vi "Set Geometry.vi"(0 "reference in":refnum<class "Manipulator.lvclass">, 5 "Lengths.a":dbl, 7 "Lengths.b":dbl, 9 "Lengths.c":dbl, 11 "error in (no error)":errorcluster) -> (4 "reference out":refnum<class "Manipulator.lvclass">, 15 "error out":errorcluster)   [LabVIEW 2014, in "Manipulator.lvclass"]
uses:
  Manipulator.lvclass
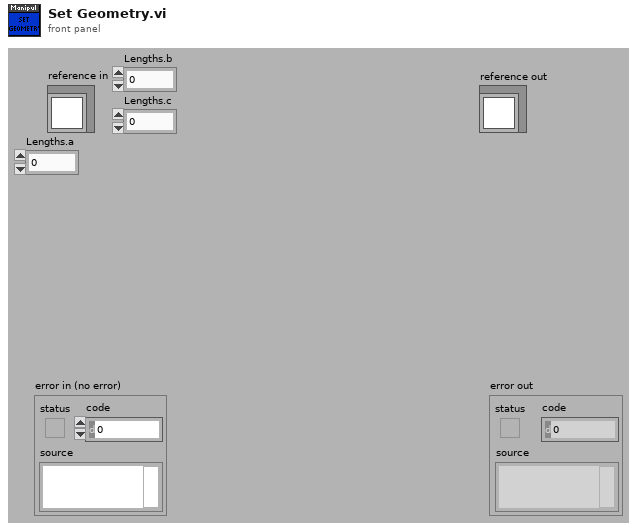
[diagram p1: front panel]
types:
  T1 = typedef "Manipulator.lvclass/ObjectAttributes.ctl" = cluster{"Coordinates":cluster{"X":dbl, "Y":dbl, "Z":dbl}, "Angles":cluster{"THETA_1":dbl, "THETA_2":dbl, "THETA_3":dbl, "THETA_4":dbl, "THETA_5":dbl, "THETA_6":dbl, "THETA_7":dbl, "THETA_8":dbl, "THETA_9":dbl, "THETA_10":dbl}, "Lengths":cluster{"a":dbl, "b":dbl, "c":dbl, "d":dbl, "e":dbl}, "Coordinates of joints":cluster{"A":cluster{"X":dbl, "Y":dbl, "Z":dbl}, "B":cluster{"X":dbl, "Y":dbl, "Z":dbl}, "C":cluster{"X":dbl, "Y":dbl, "Z":dbl}, "D":cluster{"X":dbl, "Y":dbl, "Z":dbl}}}
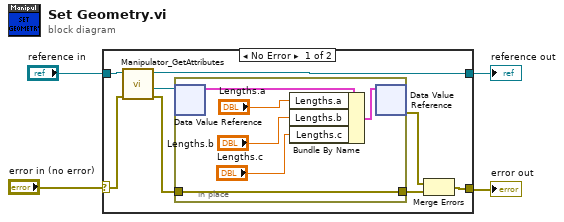
[diagram p0: block diagram]
diagram:
  n1 = case shown="No Error" "error in (no error)" {
    selector: "error in (no error)" -> [w7 w20]
    tunnel: [w11 w20] -> w3
    tunnel: [w9 w19] -> w1
    tunnel: "reference in" -> [w10 w19]
    frame No Error {
      n2 = call "Manipulator_GetAttributes.vi"("error in (no error)"=w7, "reference in"=w10) -> ("error out"=w6:errorcluster, "DataRef"=w8:refnum<data-value>, "reference out"=w9:refnum<class "Manipulator.lvclass">)  [unwired: 6 in, 1 out]
      n3 = in-place {
        in-place-border: w6 -> [w17]
        in-place-border: [w17] -> w5
        n4 = in-place-dvr #1(w8) -> (w16:T1)  [unwired: 1 out]
        n5 = Bundle By Name(cluster=w16, "Lengths.a"="Lengths.a", "Lengths.b"="Lengths.b", "Lengths.c"="Lengths.c") -> (w18:T1)
        n6 = in-place-dvr #1(w18) -> (w12:errorcluster)  [unwired: 1 out]
      }
      n7 = Merge Errors(w12, w5) -> (w11:errorcluster)
    }
    frame Error {
    }
  }
  "error out" <- w3
  "reference out" <- w1
